vi "Read Configuration Typedef.vi"() -> ()   [LabVIEW 2016, in "LVOOP Introduction.lvlib"]
doc: "Illustrates how to read a configuration settings file using typedefinitions.\n\nLizenziert unter EUPL V. 1.1"
uses:
  LVOOP Introduction.lvlib
  Typedefs/Configuration.ctl
  Typedefs/Section 1.ctl
  Typedefs/Section 2.ctl
  <vilib>/Utility/config.llb/Read Key (Boolean).vi
  <vilib>/Utility/config.llb/Read Key (Double).vi
  <vilib>/Utility/config.llb/Read Key (Path).vi
  <vilib>/Utility/config.llb/Read Key (String).vi
  <vilib>/Utility/config.llb/NI_LVConfig.lvlib
panel:
  in  "configuration file path":path
  out "Configuration":T1
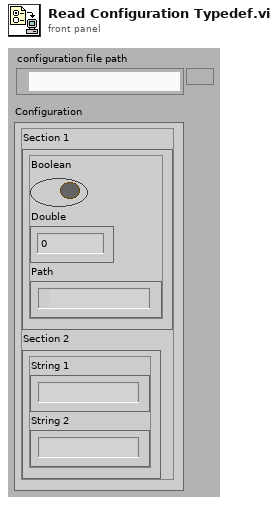
[diagram p1: front panel]
types:
  T1 = typedef "LVOOP Introduction.lvlib/Configuration.ctl" = cluster{"Section 1":T2, "Section 2":T3}
  T2 = typedef "LVOOP Introduction.lvlib/Section 1.ctl" = cluster{"Boolean":bool, "Double":dbl, "Path":path}
  T3 = typedef "LVOOP Introduction.lvlib/Section 2.ctl" = cluster{"String 1":string, "String 2":string}
  T4 = typedef "NI_LVConfig.lvlib/Config Data RefNum.ctl" = refnum<k1>
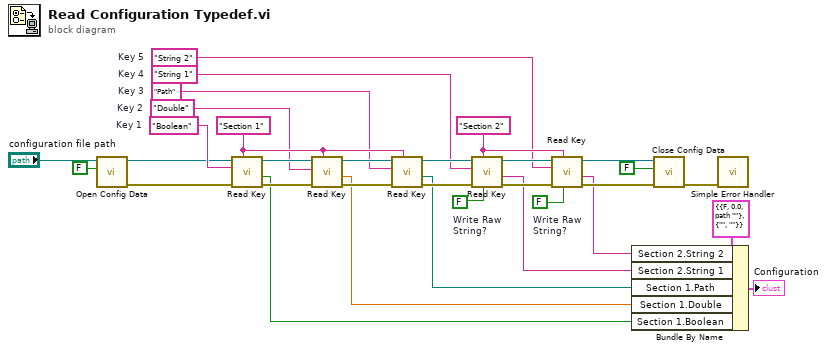
[diagram p0: block diagram]
diagram:
  w11 = FALSE  # Write Raw String?
  w12 = FALSE  # Write Raw String?
  w16 = "String 2"  # Key 5
  w17 = "String 1"  # Key 4
  w18 = "Path"  # Key 3
  w19 = "Double"  # Key 2
  w20 = "Boolean"  # Key 1
  w21 = "Section 2" ("section")
  w22 = "Section 1" ("section")
  n1 = call <vilib>:"Open Config Data.vi"("create file if necessary (T)"=FALSE ("create file if necessary? (T)"), "configuration file path"="configuration file path") -> ("error out"=w14:errorcluster, "refnum"=w13:T4)  [unwired: 7 in, 1 out]
  n2 = call-poly <vilib>:"Read Key.vi"("section"=w22, "error in (no error)"=w14, "key"=w20, "refnum"=w13) -> ("error out"=w32:errorcluster, "value"=w3:bool, "refnum out"=w30:T4)  [unwired: 1 in, 4 out]
  n3 = call-poly <vilib>:"Read Key.vi"("section"=w22, "error in (no error)"=w32, "key"=w19, "refnum"=w30) -> ("error out"=w27:errorcluster, "value"=w4:dbl, "refnum out"=w28:T4)  [unwired: 1 in, 4 out]
  n4 = call-poly <vilib>:"Read Key.vi"("section"=w22, "error in (no error)"=w27, "key"=w18, "refnum"=w28) -> ("error out"=w31:errorcluster, "value"=w5:path, "refnum out"=w29:T4)  [unwired: 1 in, 4 out]
  n5 = call-poly <vilib>:"Read Key.vi"("read raw string? (F)"=w11, "section"=w21, "error in (no error)"=w31, "key"=w17, "refnum"=w29) -> ("error out"=w24:errorcluster, "value"=w6:string, "refnum out"=w23:T4)  [unwired: 1 in, 3 out]
  n6 = call-poly <vilib>:"Read Key.vi"("read raw string? (F)"=w12, "section"=w21, "error in (no error)"=w24, "key"=w16, "refnum"=w23) -> ("error out"=w26:errorcluster, "value"=w7:string, "refnum out"=w25:T4)  [unwired: 1 in, 3 out]
  n7 = Bundle By Name(cluster=T1 {"Section 1"={"Boolean"=FALSE, "Double"=0.0, "Path"=path ""}, "Section 2"={"String 1"="", "String 2"=""}} ("Configuration"), "Section 2.String 2"=w7, "Section 2.String 1"=w6, "Section 1.Path"=w5, "Section 1.Double"=w4, "Section 1.Boolean"=w3) -> (→"Configuration":T1)
  n8 = call <vilib>:"Close Config Data.vi"("error in (no error)"=w26, "write file if changed (T)"=FALSE ("write configuration file? (T)"), "refnum"=w25) -> ("error out"=w15:errorcluster)  [unwired: 8 out]
  n9 = call <vilib>:"Simple Error Handler.vi"("error in (no error)"=w15) -> ()  [unwired: 1 in, 8 out]
